vi "RichToFlatcif_manager_SystemStatus.vi"(5 "OutputClusterType":T1, 11 "InputCluster":T5) -> (3 "OutputCluster":T1)   [LabVIEW 2021, in "CIF_Launcher_server.lvlib"]
uses:
  CIF_Launcher_server.lvlib
  cif_manager_SystemStatus.ctl
  cif_manager_ClockConversionArray.ctl
  cif_manager_ClockConversion.ctl
  cif_manager_TimePair.ctl
  cif_manager_SystemStatus_Flat.ctl
  cif_manager_ClockConversionArray_Flat.ctl
  cif_manager_ClockConversion_Flat.ctl
  cif_manager_TimePair_Flat.ctl
  RichToFlatcif_manager_ClockConversion.vi
  RichToFlatcif_manager_TimePair.vi
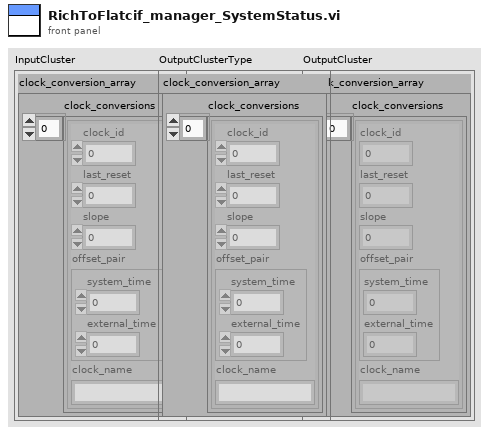
[diagram p1: front panel]
types:
  T1 = typedef "CIF_Launcher_server.lvlib/cif_manager_SystemStatus_Flat.ctl" = cluster{"clock_conversion_array":T2}
  T2 = typedef "CIF_Launcher_server.lvlib/cif_manager_ClockConversionArray_Flat.ctl" = cluster{"clock_conversions":T3[]}
  T3 = typedef "CIF_Launcher_server.lvlib/cif_manager_ClockConversion_Flat.ctl" = cluster{"clock_id":u32, "last_reset":i64, "slope":dbl, "offset_pair":T4, "clock_name":string}
  T4 = typedef "CIF_Launcher_server.lvlib/cif_manager_TimePair_Flat.ctl" = cluster{"system_time":i64, "external_time":i64}
  T5 = typedef "CIF_Launcher_server.lvlib/cif_manager_SystemStatus.ctl" = cluster{"clock_conversion_array":T6}
  T6 = typedef "CIF_Launcher_server.lvlib/cif_manager_ClockConversionArray.ctl" = cluster{"clock_conversions":T7[]}
  T7 = typedef "CIF_Launcher_server.lvlib/cif_manager_ClockConversion.ctl" = cluster{"clock_id":u32, "last_reset":i64, "slope":dbl, "offset_pair":T8, "clock_name":string}
  T8 = typedef "CIF_Launcher_server.lvlib/cif_manager_TimePair.ctl" = cluster{"system_time":i64, "external_time":i64}
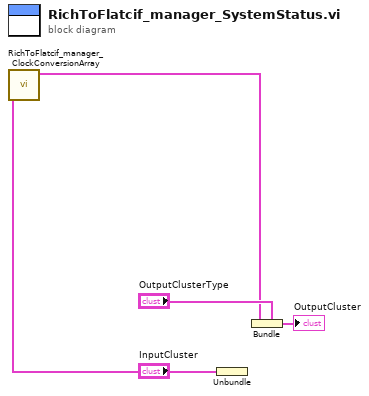
[diagram p0: block diagram]
diagram:
  n1 = Unbundle "Unbundle"("InputCluster") -> ("clock_conversion_array"=w2:T6)
  n2 = call "RichToFlatcif_manager_ClockConversionArray.vi"("InputCluster"=w2) -> ("OutputCluster"=w1:T2)  [unwired: 10 in]
  n3 = Bundle "Bundle"(cluster="OutputClusterType", "clock_conversion_array"=w1) -> (→"OutputCluster":T1)
